vi "Create Scheduled MessaGE.vi"(8 "error in":errorcluster, 11 "1553 Scheduled Message Configuration in":T1) -> (0 "error out":errorcluster, 3 "message out":refnum<k24>)   [LabVIEW 2020, in "Ballard_1553_Hardware_ni.lvlib"]
uses:
  Ballard_1553_Hardware_ni.lvlib
  C:/Users/Administrator/Desktop/GIT/Ballard-MIL-STD-1553-Custom-Device/Source/System Explorer/SubVIs/Parse XML Ballard/1.2/BTIXML_SerDes.dll
  Ballard-MIL-STD-1553-Custom-Device/Source/System Explorer/SubVIs/Parse XML Ballard/1.2/BTIXML_SerDes.dll
  _typedefs/schedItem1553_type.ctl
  _typedefs/frame_entry_type.ctl
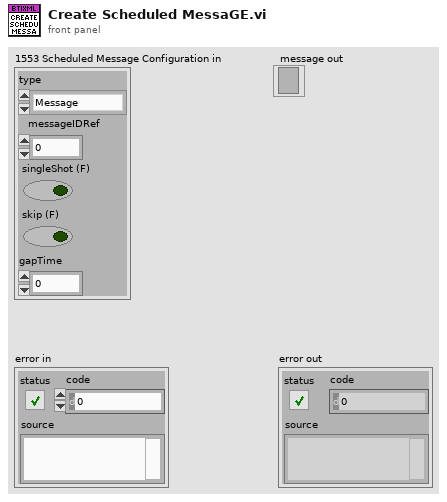
[diagram p1: front panel]
types:
  T1 = typedef "Ballard_1553_Hardware_ni.lvlib/schedItem1553_type.ctl" = cluster{"type":T2, "messageIDRef":i32, "singleShot (F)":bool, "skip (F)":bool, "gapTime":dbl}
  T2 = typedef "Ballard_1553_Hardware_ni.lvlib/frame_entry_type.ctl" = enum16{"Message", "Gap", "Pulse", "Log", "Pause", "Restart", "Halt"}
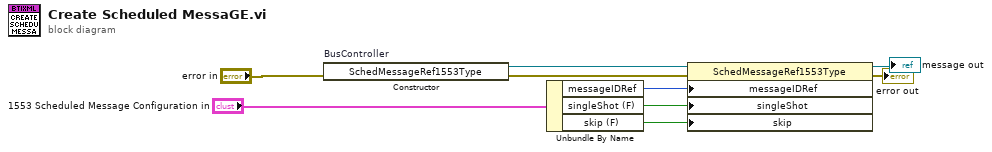
[diagram p0: block diagram]
diagram:
  n1 = constructor on="BusController" class="SchedMessageRef1553Type"(error in="error in") -> (reference out=w4:refnum<k24>, error out=w3:errorcluster)  [unwired: 2 in, 1 out]
  n2 = Unbundle By Name("1553 Scheduled Message Configuration in") -> ("messageIDRef"=w5:i32, "singleShot (F)"=w6:bool, "skip (F)"=w7:bool)
  n3 = property class="SchedMessageRef1553Type"(reference=w4, error in=w3, "messageIDRef"=w5, "singleShot"=w6, "skip"=w7) -> (reference out=→"message out":refnum<k24>, error out=→"error out":errorcluster)
